vi "Word Statistics by Letter.vi"(11 "Dictionary":string[](array[string])) -> (3 "Word Statistic":T1[](array[typedef]))   [LabVIEW 2015]
uses:
  TypeDef/Word Statistic.ctl
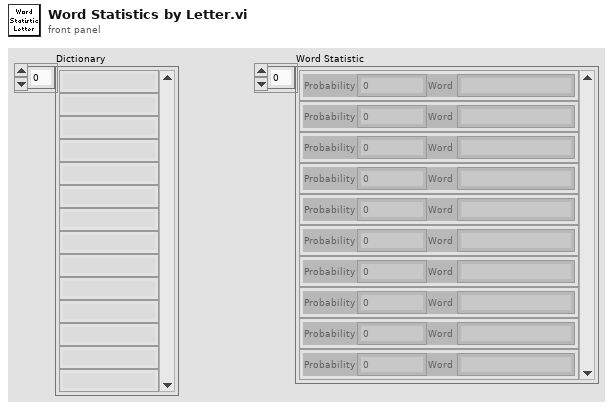
[diagram p1: front panel]
types:
  T1 = typedef "Word Statistic.ctl" = cluster{"Probability":dbl, "Word":string}
  T2 = typedef "Letter Statistic.ctl" = cluster{"Letter":string, "any":dbl, "1":dbl, "2":dbl, "3":dbl, "4":dbl, "5":dbl}
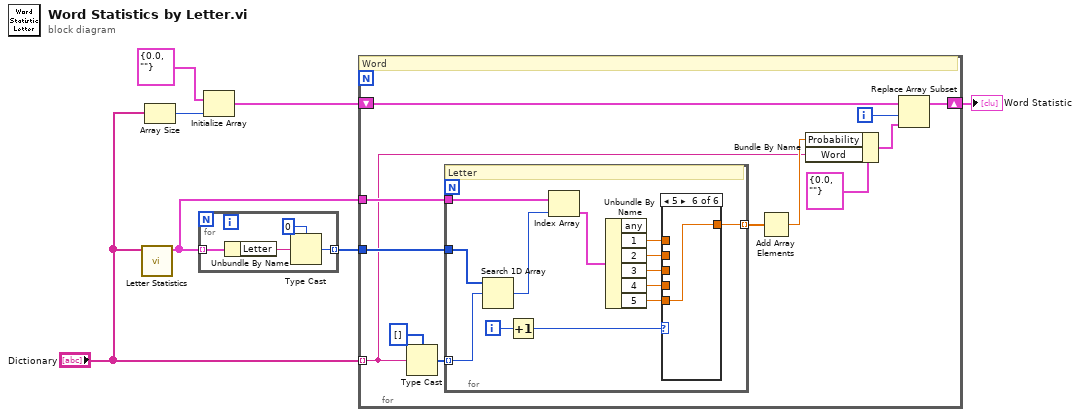
[diagram p0: block diagram]
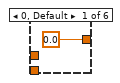
[diagram p2: hidden frame]
diagram:
  n1 = call "Letter Statistics.vi"("Dictionary"="Dictionary") -> ("Statistic"=w6:T2[])  [unwired: 10 in]
  n2 = Array Size(array="Dictionary") -> (size(s)=w4:i32)
  n3 = for {
    tunnel: w6 -> [w11] mode=indexing
    tunnel: [w9] -> w7 mode=indexing
    n4 = Unbundle By Name(w11) -> ("Letter"=w8:string)
    n5 = Type Cast(type=u8 0, x=w8) -> (*(type *) &x=w9:u8)
  }
  n6 = Initialize Array(T1 {"Probability"=0.0, "Word"=""} ("Word Statistic"), w4) -> (w2:T1[])
  n7 = for {
    tunnel: "Dictionary" -> [w12] mode=indexing
    tunnel: w6 -> [w23]
    tunnel: w7 -> [w22]
    shift-right: [w17] -> w1
    shift-left: w2 -> [w18]
    i -> [w15]
    # "Word"
    n8 = Type Cast(type=u8[] [] ("letter"), x=w12) -> (*(type *) &x=w21:u8[])
    n9 = for {
      tunnel: w21 -> [w36] mode=indexing
      tunnel: w23 -> [w32]
      tunnel: w22 -> [w31]
      tunnel: [w24] -> w14 mode=indexing
      i -> [w34]
      # "Letter"
      n10 = Search 1D Array(1D array=w31, element=w36) -> (index of element=w35:i32)  [unwired: 1 in]
      n11 = Increment(x=w34) -> (x+1=w33:i32)
      n12 = Index Array(array=w32, index=w35) -> (element=w30:T2)
      n13 = Unbundle By Name(w30) -> ("1"=w29:dbl, "2"=w28:dbl, "3"=w27:dbl, "4"=w26:dbl, "5"=w25:dbl)  [unwired: 1 out]
      n14 = case shown="5" w33 {
        tunnel: w29 -> [_ w38 _ _ _ _]
        tunnel: w28 -> [_ _ w39 _ _ _]
        tunnel: w27 -> [_ _ _ w40 _ _]
        tunnel: w26 -> [_ _ _ _ w41 _]
        tunnel: w25 -> [_ _ _ _ _ w42]
        tunnel: [0.0 w38 w39 w40 w41 w42] -> w24
        frame 0, Default {
        }
        frame 1 {
        }
        frame 2 {
        }
        frame 3 {
        }
        frame 4 {
        }
        frame 5 {
        }
      }
    }
    n15 = Add Array Elements(numeric array=w14) -> (sum=w13:dbl)
    n16 = Bundle By Name(cluster=T1 {"Probability"=0.0, "Word"=""} ("Word Statistic"), "Probability"=w13, "Word"=w12) -> (w16:T1)
    n17 = Replace Array Subset(array=w18, new element=w16, index=w15) -> (w17:T1[])
  }
  "Word Statistic" <- w1
